vi "AlliGator Generic Image Display Mouse Move Flag.vi"(1 "Image Control Refnum":T1, 2 "Flag (in)":bool, 4 "Read/Write":T2) -> (7 "Flag (out)":bool)   [LabVIEW 2021, in "AlliGator GUI.lvlib"]
doc: "Stores the selected Image Display mouse move state."
uses:
  Utilities/Read-Write.ctl
  AlliGator GUI.lvlib
  Utilities/Utilities.lvlib
  Image/Image Control Refnum.ctl
  Image/Image.lvlib
panel:
  # "see the AlliGator License on the block diagram (Ctrl+E or Window:Show Block Diagram)"
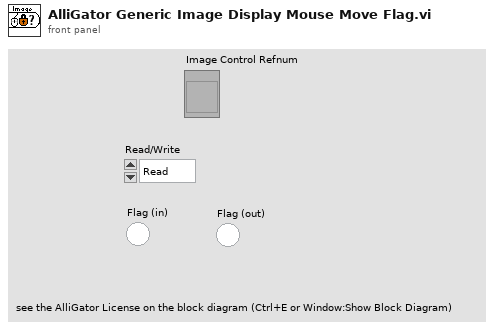
[diagram p1: front panel]
types:
  T1 = typedef "Image.lvlib/Image Control Refnum.ctl" = refnum<vi>
  T2 = typedef "Utilities.lvlib/Read-Write.ctl" = enum16{"Read", "Write"}
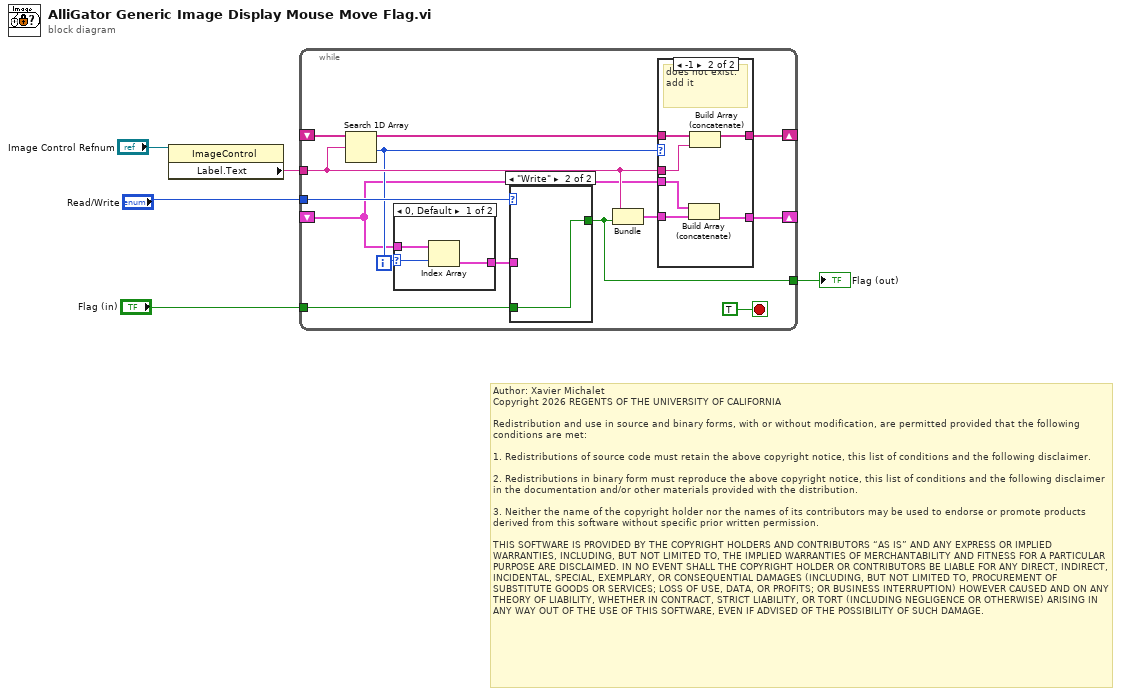
[diagram p0: block diagram]
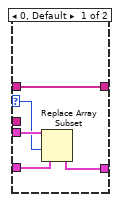
[diagram p3: hidden frame]
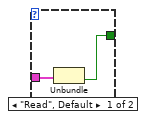
[diagram p4: hidden frame]
diagram:
  # "Author: Xavier Michalet\nCopyright 2026 REGENTS OF THE UNIVERSITY OF CALIFORNIA\n\nRedistribution and use in source and binary forms, with or without modification, are permitted provided that the following conditions are met:\n\n1. Redistributions of source code must retain the above copyright notice, this list of conditions and the following disclaimer.\n\n2. Redistributions in binary form must reproduce the above copyright notice, this list of conditions and the following disclaimer in the documentation and/or other materials provided with the distribution.\n\n3. Neither the name of the copyright holder nor the names of its contributors may be used to endorse or promote products derived from this software without specific prior written permission.\n\nTHIS SOFTWARE IS PROVIDED BY THE COPYRIGHT HOLDERS AND CONTRIBUTORS “AS IS” AND ANY EXPRESS OR IMPLIED WARRANTIES, INCLUDING, BUT NOT LIMITED TO, THE IMPLIED WARRANTIES OF MERCHANTABILITY AND FITNESS FOR A PARTICULAR PURPOSE ARE DISCLAIMED. IN NO EVENT SHALL THE COPYRIGHT HOLDER OR CONTRIBUTORS BE LIABLE FOR ANY DIRECT, INDIRECT, INCIDENTAL, SPECIAL, EXEMPLARY, OR CONSEQUENTIAL DAMAGES (INCLUDING, BUT NOT LIMITED TO, PROCUREMENT OF SUBSTITUTE GOODS OR SERVICES; LOSS OF USE, DATA, OR PROFITS; OR BUSINESS INTERRUPTION) HOWEVER CAUSED AND ON ANY THEORY OF LIABILITY, WHETHER IN CONTRACT, STRICT LIABILITY, OR TORT (INCLUDING NEGLIGENCE OR OTHERWISE) ARISING IN ANY WAY OUT OF THE USE OF THIS SOFTWARE, EVEN IF ADVISED OF THE POSSIBILITY OF SUCH DAMAGE."
  n1 = property class="ImageControl"(reference="Image Control Refnum") -> ("Label.Text"=w2:string)  [unwired: 1 in, 2 out]
  n2 = while {
    tunnel: "Read/Write" -> [w16]
    shift-right: [w10] -> _
    shift-left: _ -> [w7]
    tunnel: "Flag (in)" -> [w8]
    tunnel: w2 -> [w14]
    tunnel: [w15] -> w1
    shift-right: [w12] -> _
    shift-left: _ -> [w13]
    stop <- TRUE stop-if-true
    n3 = Search 1D Array(1D array=w13, element=w14) -> (index of element=w9:i32)  [unwired: 1 in]
    n4 = case shown="0, Default" w9 {
      selector: w9 -> [w19 _]
      tunnel: w7 -> [w20 _]
      tunnel: [w18 _] -> w6
      frame 0, Default {
        n5 = Index Array(array=w20, index=w19) -> (element=w18:cluster{"Label.Text":string, "Flag (in)":bool})
      }
      frame -1 {
      }
    }
    n6 = case shown="\"Write\"" w16 {
      tunnel: [w32 w34] -> w15
      tunnel: w8 -> [_ w34]
      tunnel: w6 -> [w33 _]
      frame "Read", Default {
        n7 = Unbundle(w33) -> ("Flag (in)"=w32:bool)  [unwired: 1 out]
      }
      frame "Write" {
      }
    }
    n8 = Bundle("Label.Text"=w14, "Flag (in)"=w15) -> (w11:cluster{"Label.Text":string, "Flag (in)":bool})  [unwired: 1 in]
    n9 = case shown="-1" w9 {
      selector: w9 -> [w21 _]
      tunnel: w14 -> [_ w29]
      tunnel: w13 -> [w25 w31]
      tunnel: [w25 w30] -> w12
      tunnel: w11 -> [w23 w28]
      tunnel: [w22 w27] -> w10
      tunnel: w7 -> [w24 w26]
      frame 0, Default {
        n10 = Replace Array Subset(array=w24, new element=w23, index=w21) -> (w22:cluster{"Label.Text":string, "Flag (in)":bool}[])
      }
      frame -1 {
        # "does not exist: add it"
        n11 = Build Array (concatenate)(w26, w28) -> (w27:cluster{"Label.Text":string, "Flag (in)":bool}[])
        n12 = Build Array (concatenate)(w31, w29) -> (w30:string[])
      }
    }
  }
  "Flag (out)" <- w1
